vi "BezahlSimulation.vi"(8 "error in (no error)":errorcluster, 10 "Preis":dbl) -> (0 "error out":errorcluster, 2 "Betrag erreicht":bool)   [LabVIEW 2023]
doc: "Bezahlsimulation\nerstellt: DI FH Mst Werner Bischof\nDatum: 22.10.2025"
panel:
  out "Restgeldausgabe":dbl
  in  "Storno":bool
  out "Guthaben":dbl
  in  "100Euro":bool
  in  "50Euro":bool
  in  "20Euro":bool
  in  "10Euro":bool
  in  "5Euro":bool
  in  "2Euro":bool
  in  "Bezahlen":bool
  in  "1Euro":bool
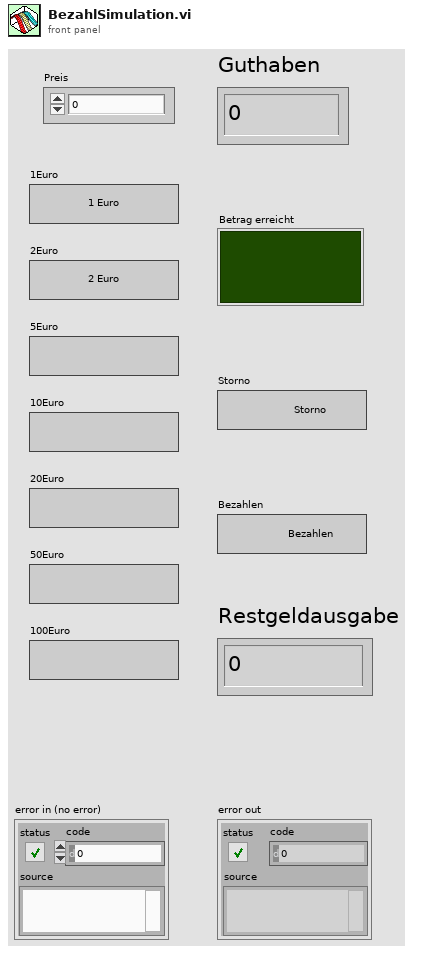
[diagram p1: front panel]
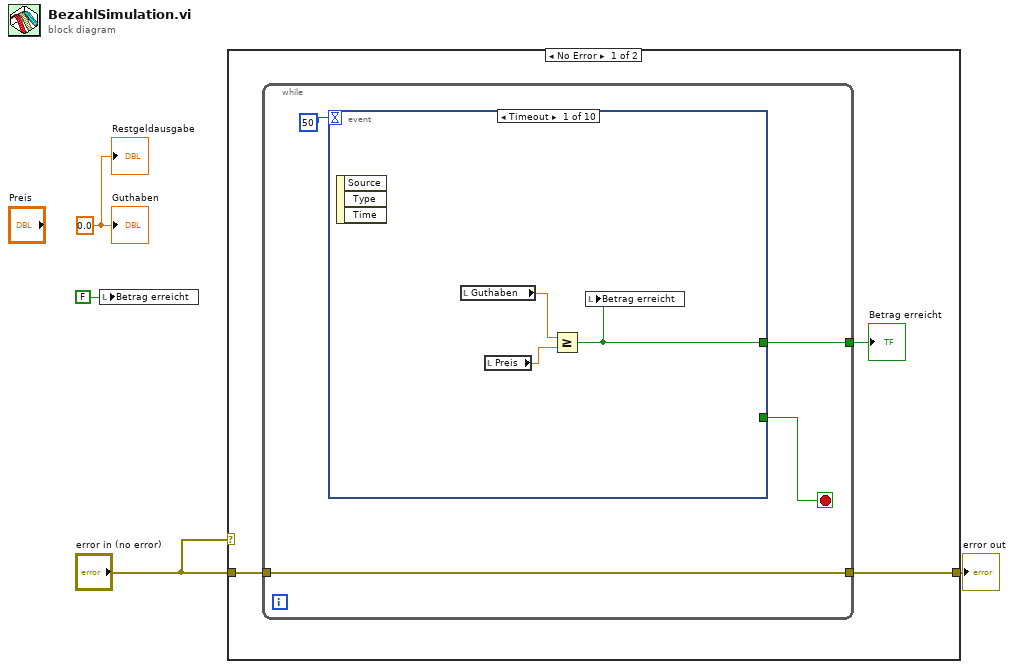
[diagram p0: block diagram]
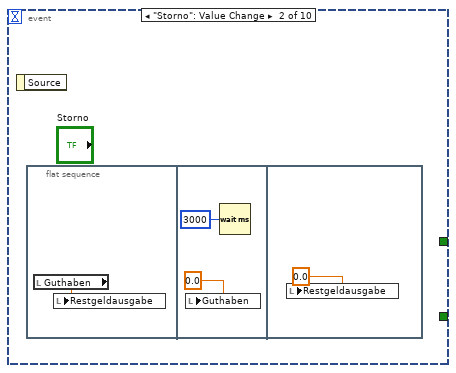
[diagram p2: hidden frame]
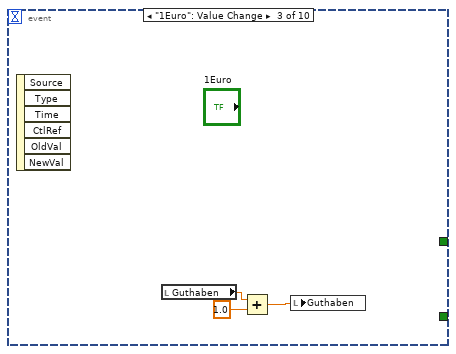
[diagram p3: hidden frame]
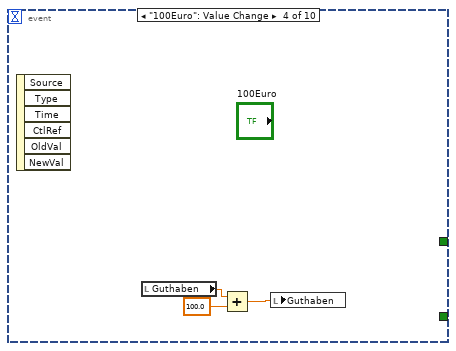
[diagram p4: hidden frame]
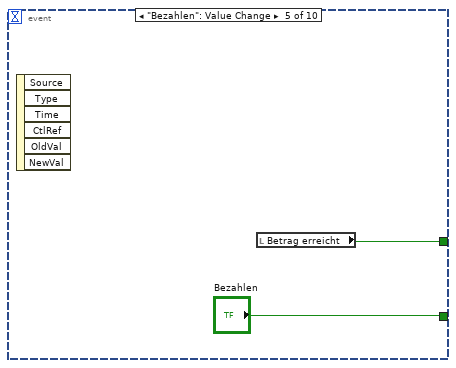
[diagram p5: hidden frame]
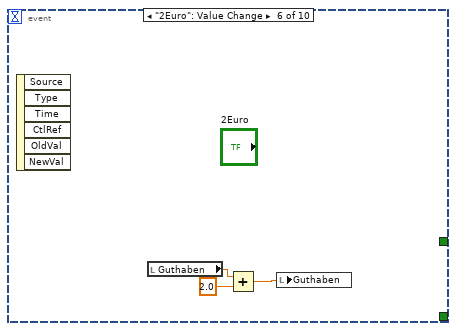
[diagram p6: hidden frame]
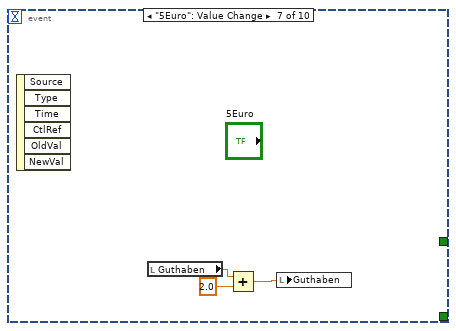
[diagram p7: hidden frame]
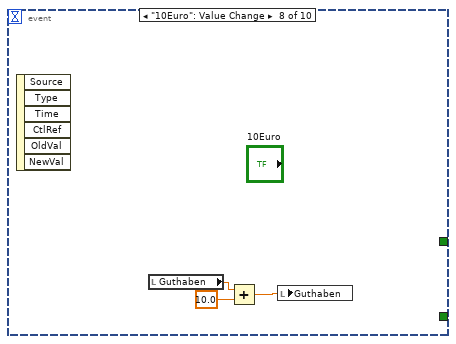
[diagram p8: hidden frame]
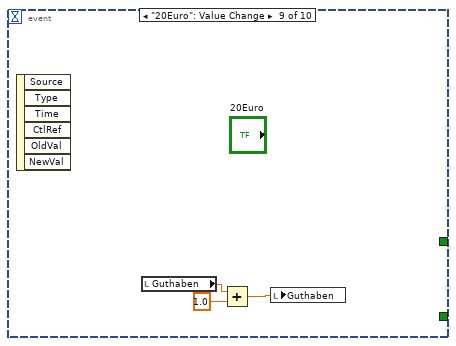
[diagram p9: hidden frame]
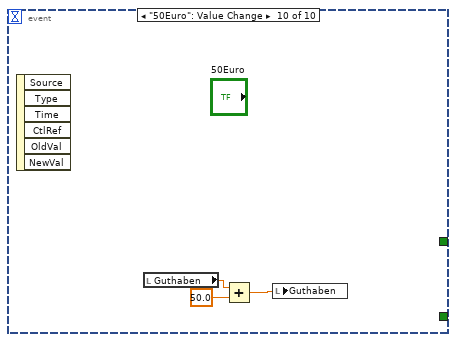
[diagram p10: hidden frame]
diagram:
  w3 = 0.0 ("Guthaben")
  n1 = local write "Betrag erreicht"(FALSE ("Betrag erreicht")) -> ()
  n2 = case shown="No Error" "error in (no error)" {
    tunnel: "error in (no error)" -> [w7 w42]
    tunnel: [w6 w42] -> w2
    frame No Error {
      n3 = while {
        tunnel: [w9] -> w5
        tunnel: w7 -> [w8]
        tunnel: [w8] -> w6
        stop <- w11 stop-if-true
        n4 = event shown="[0] Timeout" {
          selector: _ -> [_ _ _ _ _ _ _ _ _ _]
          dyn-events: _ -> [_ _ _ _ _ _ _ _ _ _]
          timeout: 50 -> [_ _ _ _ _ _ _ _ _ _]
          tunnel: [_ _ _ _ "Bezahlen" _ _ _ _ _] -> w11
          tunnel: [w12 _ _ _ w25 _ _ _ _ _] -> w9
          event Timeout {
            n5 = event-data() -> ()  [unwired: 1 in, 3 out]
            n6 = local read "Guthaben"() -> (w14:dbl)
            n7 = local read "Preis"() -> (w13:dbl)
            n8 = Greater Or Equal?(x=w14, y=w13) -> (x >= y?=w12:bool)
            n9 = local write "Betrag erreicht"(w12) -> ()
          }
          event "Storno": Value Change {
            n10 = event-data() -> ()  [unwired: 1 in, 1 out]
            n11 = flat-sequence {
              frame #0 {
                n12 = local read "Guthaben"() -> (w15:dbl)
                n13 = local write "Restgeldausgabe"(w15) -> ()
              }
              frame #1 {
                n14 = local write "Guthaben"(0.0 ("Guthaben")) -> ()
                n15 = Wait (ms)(milliseconds to wait=u32 3000) -> ()  [unwired: 1 out]
              }
              frame #2 {
                n16 = local write "Restgeldausgabe"(0.0 ("Guthaben")) -> ()
              }
            }
          }
          event "1Euro": Value Change {
            n17 = event-data() -> ()  [unwired: 1 in, 6 out]
            n18 = local read "Guthaben"() -> (w21:dbl)
            n19 = Add(x=w21, y=1.0) -> (x+y=w20:dbl)
            n20 = local write "Guthaben"(w20) -> ()
          }
          event "100Euro": Value Change {
            n21 = event-data() -> ()  [unwired: 1 in, 6 out]
            n22 = local read "Guthaben"() -> (w24:dbl)
            n23 = Add(x=w24, y=100.0) -> (x+y=w23:dbl)
            n24 = local write "Guthaben"(w23) -> ()
          }
          event "Bezahlen": Value Change {
            n25 = event-data() -> ()  [unwired: 1 in, 6 out]
            n26 = local read "Betrag erreicht"() -> (w25:bool)
          }
          event "2Euro": Value Change {
            n27 = event-data() -> ()  [unwired: 1 in, 6 out]
            n28 = local read "Guthaben"() -> (w29:dbl)
            n29 = Add(x=w29, y=2.0) -> (x+y=w28:dbl)
            n30 = local write "Guthaben"(w28) -> ()
          }
          event "5Euro": Value Change {
            n31 = event-data() -> ()  [unwired: 1 in, 6 out]
            n32 = local read "Guthaben"() -> (w32:dbl)
            n33 = Add(x=w32, y=2.0) -> (x+y=w31:dbl)
            n34 = local write "Guthaben"(w31) -> ()
          }
          event "10Euro": Value Change {
            n35 = event-data() -> ()  [unwired: 1 in, 6 out]
            n36 = local read "Guthaben"() -> (w35:dbl)
            n37 = Add(x=w35, y=10.0) -> (x+y=w34:dbl)
            n38 = local write "Guthaben"(w34) -> ()
          }
          event "20Euro": Value Change {
            n39 = event-data() -> ()  [unwired: 1 in, 6 out]
            n40 = local read "Guthaben"() -> (w38:dbl)
            n41 = Add(x=w38, y=1.0) -> (x+y=w37:dbl)
            n42 = local write "Guthaben"(w37) -> ()
          }
          event "50Euro": Value Change {
            n43 = event-data() -> ()  [unwired: 1 in, 6 out]
            n44 = local read "Guthaben"() -> (w41:dbl)
            n45 = Add(x=w41, y=50.0) -> (x+y=w40:dbl)
            n46 = local write "Guthaben"(w40) -> ()
          }
        }
      }
      "Betrag erreicht" <- w5
    }
    frame Error {
    }
  }
  "error out" <- w2
  "Guthaben" <- w3
  "Restgeldausgabe" <- w3
